vi "About Equal.vi"(1 "Standard Value":dbl format="%.2f", 2 "+/- Range":dbl format="%.2f", 3 "Input Value":dbl format="%.2f") -> (0 "In Range?":bool)   [LabVIEW 2020]
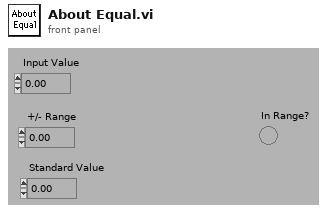
[diagram p1: front panel]
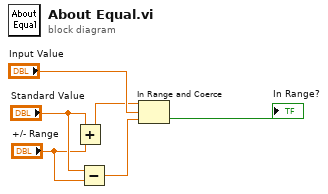
[diagram p0: block diagram]
diagram:
  n1 = Add(x="Standard Value", y="+/- Range") -> (x+y=w4:dbl)
  n2 = Subtract(x="Standard Value", y="+/- Range") -> (x-y=w1:dbl)
  n3 = In Range and Coerce(upper limit=w4, x="Input Value", lower limit=w1) -> (In Range?=→"In Range?":bool)  [unwired: 1 out]
